vi "Python Node test.vi"() -> ()   [LabVIEW 2019]
uses:
  GlobalVars.vi
panel:
  out "return value":cluster{i32[], i32[], i32[], string[][]}
  out "xt end":i32
  out "xt length":i32
  out "xt and port lists match?":bool
  in  "batch file":path
  in  "python module path":path
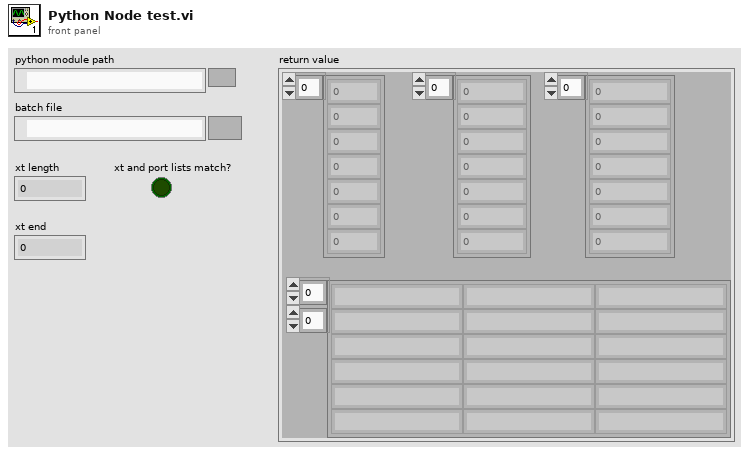
[diagram p1: front panel]
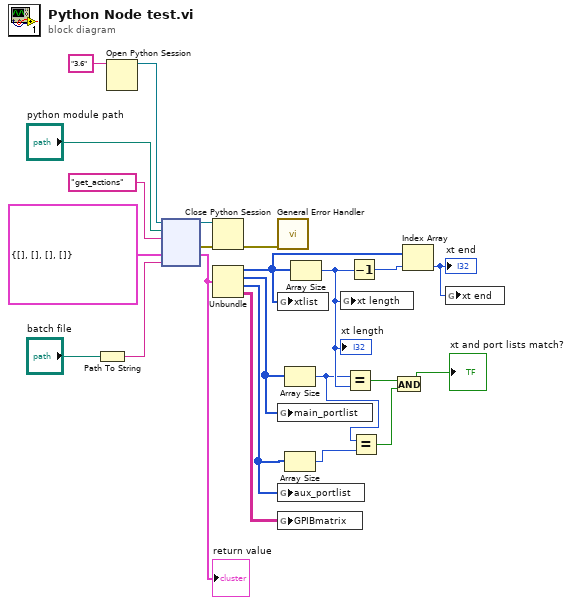
[diagram p0: block diagram]
diagram:
  n1 = Path To String(path="batch file") -> (string=w15:string)
  n2 = Open Python Session(python version="3.6" ("Python version")) -> (session out=w22:refnum<k35>)  [unwired: 2 in, 1 out]
  n3 = node(w22, "python module path", "get_actions" ("get"), cluster{i32[], i32[], i32[], string[][]} {[], [], [], []}, w15) -> (w17:refnum<k35>, w10:errorcluster, w11:cluster{i32[], i32[], i32[], string[][]})  [unwired: 2 in, 2 out]
  "return value" <- w11
  n4 = Close Python Session(session in=w17, error in=w10) -> (11:w19:errorcluster)
  n5 = Unbundle(w11) -> (w8:i32[], w9:i32[], w4:i32[], w7:string[][])
  n6 = call <vilib>:"General Error Handler.vi"("error in (no error)"=w19) -> ()  [unwired: 10 in, 5 out]
  n7 = global write "GlobalVars.vi" "xtlist"(w8) -> ()
  n8 = global write "GlobalVars.vi" "main_portlist"(w9) -> ()
  n9 = global write "GlobalVars.vi" "aux_portlist"(w4) -> ()
  n10 = global write "GlobalVars.vi" "GPIBmatrix"(w7) -> ()
  n11 = Array Size(array=w9) -> (size(s)=w2:i32)
  n12 = Array Size(array=w4) -> (size(s)=w3:i32)
  n13 = Array Size(array=w8) -> (size(s)=w13:i32)
  "xt length" <- w13
  n14 = global write "GlobalVars.vi" "xt length"(w13) -> ()
  n15 = Equal?(x=w2, y=w13) -> (x = y?=w14:bool)
  n16 = Decrement(x=w13) -> (x-1=w12:i32)
  n17 = Equal?(x=w2, y=w3) -> (x = y?=w1:bool)
  n18 = And(x=w14, y=w1) -> (x .and. y?=→"xt and port lists match?":bool)
  n19 = Index Array(array=w8, index=w12) -> (element=w6:i32)
  "xt end" <- w6
  n20 = global write "GlobalVars.vi" "xt end"(w6) -> ()
